vi "GA Get Axis Enc Pos.vi"(7 "pClock":u32, 8 "error in (no error)":errorcluster caption="错误输入（无错误）", 9 "nCount":i16, 10 "pValue":dbl, 11 "nAxisNum":i16) -> (0 "error out":errorcluster caption="错误输出", 2 "pValue out":dbl, 3 "function return":i32, 5 "pClock out":u32)   [LabVIEW 2024, in "GAS.lvlib"]
doc: "extern \"C\" __declspec(dllimport) int GA_GetAxisEncPos(short nAxisNum,double *pValue,short nCount=1,unsigned long *pClock=NULL);"
uses:
  GAS.lvlib
  GAS.dll
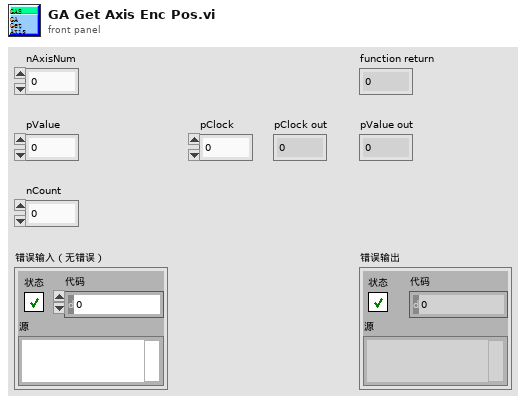
[diagram p1: front panel]
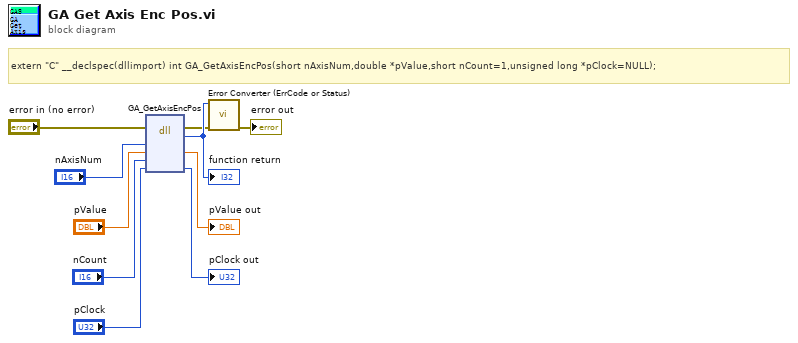
[diagram p0: block diagram]
diagram:
  # "extern \"C\" __declspec(dllimport) int GA_GetAxisEncPos(short nAxisNum,double *pValue,short nCount=1,unsigned long *pClock=NULL);"
  n1 = dll-call lib="PTH2?abs D实验室软件（勿删）集成测试系统GAS.*" fn="GA_GetAxisEncPos"(error in="error in (no error)", "nAxisNum"="nAxisNum", "pValue"="pValue", "nCount"="nCount", "pClock"="pClock") -> (error out=w2:errorcluster, w10:i32, "pValue"=→"pValue out":dbl, "pClock"=→"pClock out":u32)  [unwired: 4 in, 1 out]
  "function return" <- w10
  n2 = call "Error Converter (ErrCode or Status).vi"("error in (no error)"=w2, "error code"=w10) -> ("error out"=→"error out":errorcluster)  [unwired: 9 in]
